vi "Navigation.vi"   [LabVIEW 2011]
uses:
  _GlobalVariables&Libraries/ATV Program Global Variables.vi
types:
  T1 = cluster{"Navigation Coordinates":cluster{"Latitude":dbl, "Longitude":dbl}[], "Coordinate Count":u32, "Drive Speed":string, "Steer Angle":dbl, "Steering":dbl, "Direction to next Coordinate":dbl, "Drive":dbl, "Navigation Path":string}
  T2 = cluster{"End ATV Program":bool, "E-Stop":bool, "Save Logfile":bool, "Logfile Iteration Delay (ms)":u32, "Loop iteration time (ms)":u32, "Logfile Location":path, "Default GPS Navigation Path":path, "Computer":string, "Default GPS Boundary Path":path}
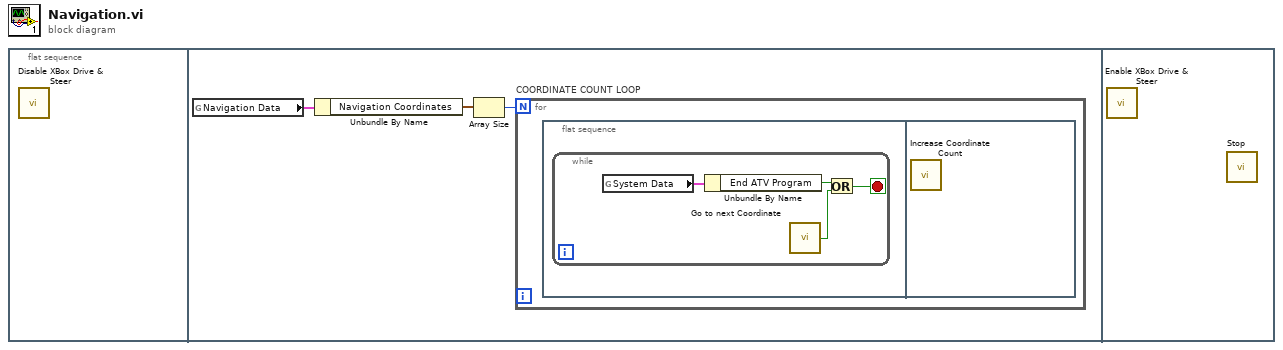
[diagram p0: block diagram]
diagram:
  n1 = flat-sequence {
    frame #0 {
      n2 = call "Disable XBox Drive & Steer.vi"() -> ()  [unwired: 12 in]
    }
    frame #1 {
      n3 = global read "ATV Program Global Variables.vi" "Navigation Data"() -> (w3:T1)
      n4 = Unbundle By Name(w3) -> ("Navigation Coordinates"=w2:cluster{"Latitude":dbl, "Longitude":dbl}[])
      n5 = Array Size(array=w2) -> (size(s)=w1:i32)
      n6 = for "COORDINATE COUNT LOOP" {
        N: w1 -> [_]
        n7 = flat-sequence {
          frame #0 {
            n8 = while {
              stop <- w4 stop-if-true
              n9 = global read "ATV Program Global Variables.vi" "System Data"() -> (w7:T2)
              n10 = Unbundle By Name(w7) -> ("End ATV Program"=w6:bool)
              n11 = call "Go to next Coordinate.vi"() -> ("Reached/Missed"=w5:bool)
              n12 = Or(x=w6, y=w5) -> (x .or. y?=w4:bool)
            }
          }
          frame #1 {
            n13 = call "Increase Coordinate Count.vi"() -> ()  [unwired: 12 in]
          }
        }
      }
    }
    frame #2 {
      n14 = call "Enable XBox Drive & Steer.vi"() -> ()  [unwired: 12 in]
      n15 = call "Stop.vi"() -> ()  [unwired: 12 in]
    }
  }
